vi "LabviewC#102.vi"() -> ()   [LabVIEW 2017]
uses:
  C:/Users/GB/Desktop/FT232H_8CHADC/FTD2XX_NET.dll
  FT232H_8CHADC/FTD2XX_NET.dll
panel:
  out "ToString 3":string
  out "ToString 2":string
  out "ToString":string
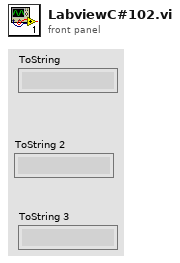
[diagram p1: front panel]
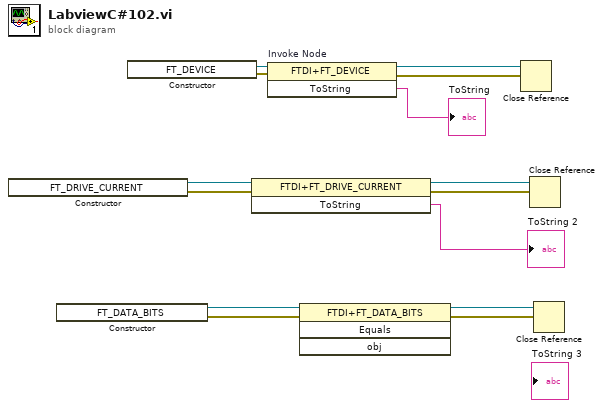
[diagram p0: block diagram]
diagram:
  n1 = constructor class="FTDI+FT_DRIVE_CURRENT"() -> (reference out=w9:refnum<k24>, error out=w7:errorcluster)  [unwired: 3 in, 1 out]
  n2 = constructor class="FTDI+FT_DATA_BITS"() -> (reference out=w4:refnum<k24>, error out=w2:errorcluster)  [unwired: 3 in, 1 out]
  n3 = constructor class="FTDI+FT_DEVICE"() -> (reference out=w14:refnum<k24>, error out=w12:errorcluster)  [unwired: 3 in, 1 out]
  n4 = invoke on="Invoke Node" class="FTDI+FT_DRIVE_CURRENT" method="ToString"(reference=w9, error in=w7) -> (reference out=w8:refnum<k24>, error out=w6:errorcluster, "ToString"=→"ToString 2":string)  [unwired: 1 in]
  n5 = invoke on="Invoke Node" class="FTDI+FT_DEVICE" method="ToString"(reference=w14, error in=w12) -> (reference out=w13:refnum<k24>, error out=w11:errorcluster, "ToString"=→"ToString":string)  [unwired: 1 in]
  n6 = invoke class="FTDI+FT_DATA_BITS" method="Equals"(reference=w4, error in=w2) -> (reference out=w3:refnum<k24>, error out=w1:errorcluster)  [unwired: 2 in, 2 out]
  n7 = Close Reference(reference=w13, error in (no error)=w11) -> ()  [unwired: 1 out]
  n8 = Close Reference(reference=w8, error in (no error)=w6) -> ()  [unwired: 1 out]
  n9 = Close Reference(reference=w3, error in (no error)=w1) -> ()  [unwired: 1 out]
